vi "Create.vi"(8 "error in (no error)":errorcluster, 11 "User Interface Events in":refnum<class "User Interface Events.lvclass">) -> (0 "error out":errorcluster, 3 "User Interface Events out":refnum<class "User Interface Events.lvclass">)   [LabVIEW 2019, in "DSF Core.lvlib" / "User Interface Events.lvclass"]
uses:
  User Interface Events.lvclass
  User Interface Events.lvclass/User Interface Events.ctl
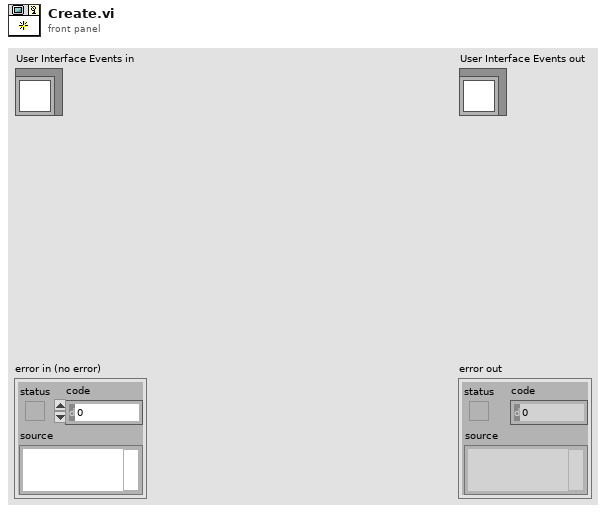
[diagram p1: front panel]
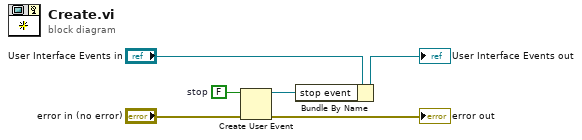
[diagram p0: block diagram]
diagram:
  w4 = FALSE  # stop
  n1 = Create User Event(user event datatype=w4, error in="error in (no error)") -> (user event=w3:refnum<user-event>, error out=→"error out":errorcluster)
  n2 = Bundle By Name(cluster="User Interface Events in", "stop event"=w3) -> (→"User Interface Events out":refnum<class "User Interface Events.lvclass">)
